vi "database1查询.vi"(6 "时间2":string, 7 "error in (no error)":errorcluster, 8 "table":string, 9 "时间1":string, 10 "database":string="database1.mdb") -> (0 "error out":errorcluster, 2 "data":string[][](table), 3 "recordset data":variant[][](array[variant]))   [LabVIEW 2016, in "数据传输系统.lvlib"]
uses:
  <vilib>/Utility/sysdir.llb/System Directory Type.ctl
  <vilib>/addons/database/Connection.llb/DB Tools Open Connec (String).vi
  <vilib>/addons/database/Connection.llb/Conn Execute.vi
  <vilib>/addons/database/Recordset.llb/Rec Fetch Recordset Data (R).vi
  <vilib>/addons/database/Recordset.llb/Rec Destroy - Connection.vi
  <vilib>/addons/database/_DB Variant To Data/Database Variant To Data.xnode
  <vilib>/addons/database/NI_Database_API.lvlib
panel:
  out "SQL query":string
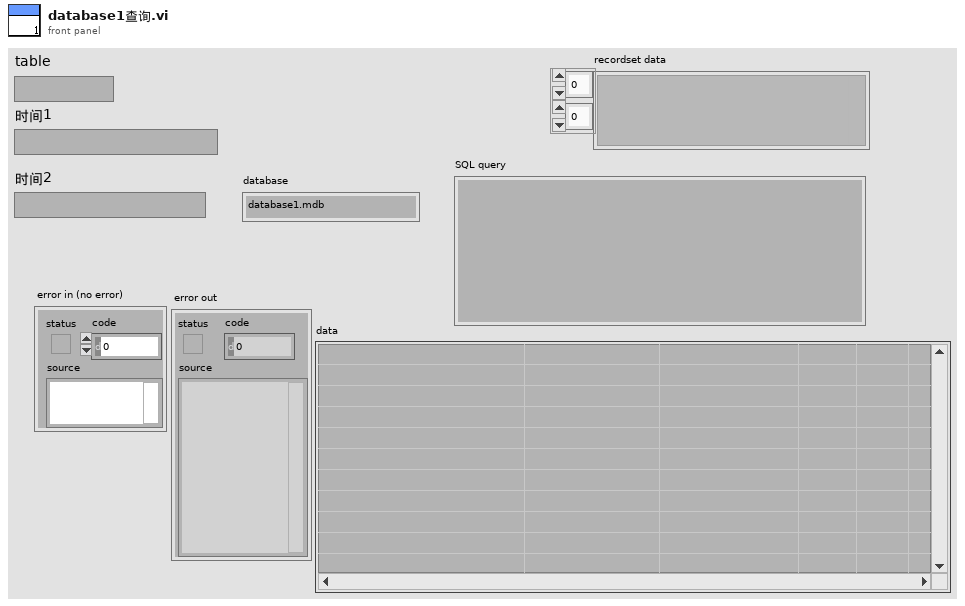
[diagram p1: front panel]
types:
  T1 = typedef "System Directory Type.ctl" = i32
  T2 = typedef "NI_Database_API.lvlib/Conn ObjectReference.ctl" = refnum<k1>
  T3 = typedef "NI_Database_API.lvlib/Rec ObjectReference.ctl" = refnum<k1>
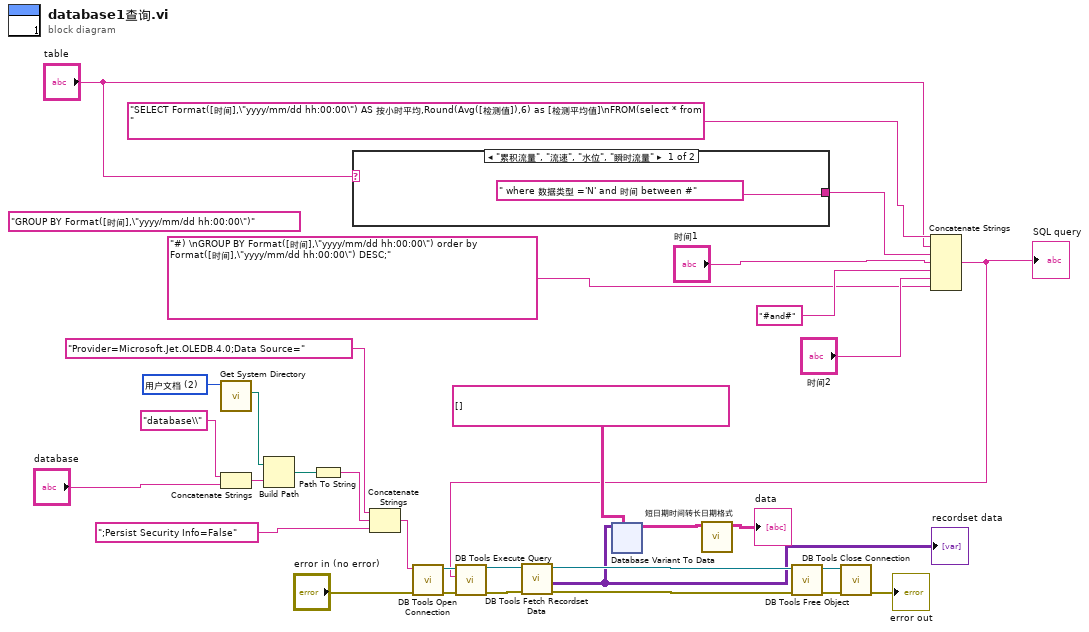
[diagram p0: block diagram]
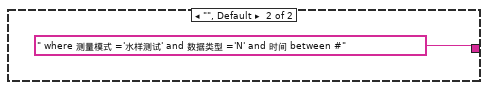
[diagram p2: hidden frame]
diagram:
  (unwired) "GROUP BY Format([时间],\"yyyy/mm/dd hh:00:00\")"
  w30 = T1 2 items=["用户目录"=0, "用户桌面"=1, "用户文档"=2, "用户应用程序数据"=3, "用户设置"=4, "用户临时目录"=5, "公共文档"=6, "公共应用程序数据"=7, "公共设置"=8, "公共缓存"=13, "系统核心库"=9, "系统安装库"=10, "应用程序文件"=11, "启动盘根目录"=12] ("system directory type")
  n1 = call <vilib>:"Get System Directory.vi"("system directory type"=w30) -> ("system directory"=w28:path)  [unwired: 10 in]
  n2 = Concatenate Strings("database\\" ("condition"), "database") -> (w22:string)
  n3 = Build Path(base path=w28, name or relative path=w22) -> (appended path=w27:path)
  n4 = Path To String(path=w27) -> (string=w26:string)
  n5 = case shown="\"累积流量\", \"流速\", \"水位\", \"瞬时流量\"" "table" {
    tunnel: [" where 数据类型 ='N' and 时间 between #" " where 测量模式 ='水样测试' and 数据类型 ='N' and 时间 between #"] -> w1
    frame "累积流量", "流速", "水位", "瞬时流量" {
    }
    frame "", Default {
    }
  }
  n6 = Concatenate Strings("Provider=Microsoft.Jet.OLEDB.4.0;Data Source=" ("condition"), w26, ";Persist Security Info=False" ("condition")) -> (w24:string)
  n7 = call-poly <vilib>:"DB Tools Open Connection.vi"("error in (no error)"="error in (no error)", "connection information"=w24) -> ("error out"=w17:errorcluster, "connection reference"=w18:T2)  [unwired: 6 in]
  n8 = Concatenate Strings("SELECT Format([时间],\"yyyy/mm/dd hh:00:00\") AS 按小时平均,Round(Avg([检测值]),6) as [检测平均值]\nFROM(select * from ", "table", w1, "时间1", "#and#", "时间2", "#) \nGROUP BY Format([时间],\"yyyy/mm/dd hh:00:00\") order by Format([时间],\"yyyy/mm/dd hh:00:00\") DESC;" ("字符串")) -> (w9:string)
  "SQL query" <- w9
  n9 = call-poly <vilib>:"DB Tools Execute Query.vi"("error in (no error)"=w17, "SQL query"=w9, "connection reference"=w18) -> ("error out"=w16:errorcluster, "recordset reference"=w13:T3)  [unwired: 5 in]
  n10 = call-poly <vilib>:"DB Tools Fetch Recordset Data.vi"("error in (no error)"=w16, "recordset reference"=w13) -> ("error out"=w19:errorcluster, "recordset data"=w12:variant[][], "recordset reference out"=w20:T3)  [unwired: 3 in]
  "recordset data" <- w12
  n11 = xnode "Database Variant To Data"("database variant"=w12, "type"=string[][] []) -> ("data"=w4:string[][])  [unwired: 1 in, 1 out]
  n12 = call "短日期时间转长日期格式.vi"("data"=w4) -> ("输出数组"=→"data":string[][])  [unwired: 10 in]
  n13 = call-poly <vilib>:"DB Tools Free Object.vi"("error in (no error)"=w19, "recordset reference"=w20) -> ("error out"=w14:errorcluster, "connection reference"=w15:T2)  [unwired: 8 in]
  n14 = call <vilib>:"DB Tools Close Connection.vi"("error in (no error)"=w14, "connection reference"=w15) -> ("error out"=→"error out":errorcluster)  [unwired: 5 in]
